vi "Ballard XML Generator.Tx Section Comment.vi"(11 "string in":string) -> (3 "string out":string)   [LabVIEW 2017]
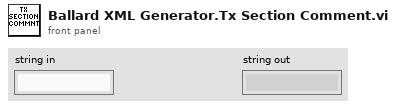
[diagram p1: front panel]
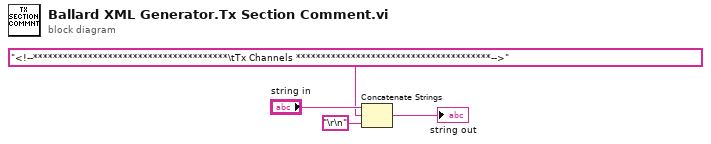
[diagram p0: block diagram]
diagram:
  n1 = Concatenate Strings("string in", "<!--***************************************\tTx Channels ***************************************-->", "\r\n") -> (→"string out":string)
